vi "DllFxpPolarToRectTemp.vi"(6 "ready for output":bool, 8 "input valid":bool, 10 "phase":fxp<+/-,64,32>, 11 "magnitude":fxp<+/-,64,32>) -> (0 "output valid":bool, 2 "y":fxp<+,1,1>, 3 "x":fxp<+,1,1>, 4 "ready for input":bool)   [LabVIEW 2017]
uses:
  <vilib>/rvi/FXPMathLib/FxpPolarToRect/subVIs/nifxpmath_PolarToRect_SimConfig.ctl
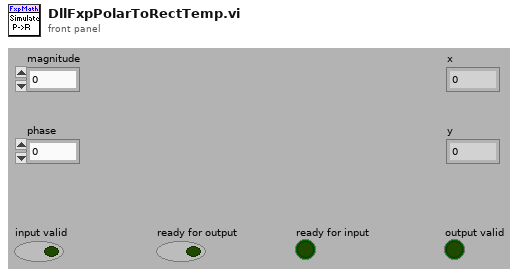
[diagram p1: front panel]
types:
  T1 = typedef "nifxpmath_PolarToRect_SimConfig.ctl" = cluster{"kXYLen":u16, "kPhaseLen":u16, "kPhaseIwl":i16, "kPhaseSigned":bool, "kMagnitudeLen":u16, "kMagnitudeSigned":bool, "kGainCompst":bool, "kCoarseRotation":bool, "kPrecision":u16, "kIteration":u16, "kQuaMode":u16, "HandShake":bool, "InputRegister":bool, "OutputRegister":bool, "CycleLimit":u16, "StrictLimit":bool, "PrescaleCycle":bool}
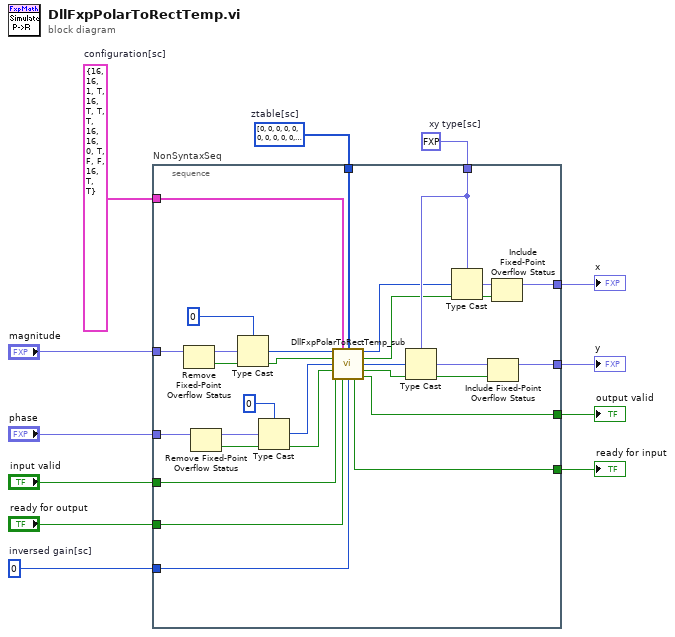
[diagram p0: block diagram]
diagram:
  w1 = T1 {"kXYLen"=16, "kPhaseLen"=16, "kPhaseIwl"=1, "kPhaseSigned"=TRUE, "kMagnitudeLen"=16, "kMagnitudeSigned"=TRUE, "kGainCompst"=TRUE, "kCoarseRotation"=TRUE, "kPrecision"=16, "kIteration"=16, "kQuaMode"=0, "HandShake"=TRUE, "InputRegister"=FALSE, "OutputRegister"=FALSE, "CycleLimit"=16, "StrictLimit"=TRUE, "PrescaleCycle"=TRUE}  # configuration[sc]
  w8 = fxp<+,1,1> 0.0  # xy type[sc]
  w9 = u64 0  # inversed gain[sc]
  w5 = u64[] [0, 0, 0, 0, 0, 0, 0, 0, 0, 0, 0, 0, 0, 0, 0, 0]  # ztable[sc]
  n1 = stacked-sequence "NonSyntaxSeq" {
    tunnel: "input valid" -> [w28]
    tunnel: w1 -> [w35]
    tunnel: "magnitude" -> [w33]
    tunnel: "phase" -> [w31]
    tunnel: w9 -> [w26]
    tunnel: w8 -> [w38]
    tunnel: [w23] -> w7
    tunnel: [w20] -> w6
    tunnel: w5 -> [w27]
    tunnel: "ready for output" -> [w25]
    tunnel: [w18] -> w3
    tunnel: [w17] -> w2
    frame #0 {
      n2 = Remove Fixed-Point Overflow Status(3:w33) -> (0:w32:bool, 1:w34:fxp<+/-,64,32>)
      n3 = Remove Fixed-Point Overflow Status(3:w31) -> (0:w29:bool, 1:w30:fxp<+/-,64,32>)
      n4 = Type Cast(type=u64 0, x=w34) -> (*(type *) &x=w16:u64)
      n5 = Type Cast(type=u64 0, x=w30) -> (*(type *) &x=w15:u64)
      n6 = call <vilib>:"DllFxpPolarToRectTemp_sub.vi"("magnitude"=w16, "configuration[sc]"=w35, "ztable"=w27, "magnitude ovfl status"=w32, "phase"=w15, "phase ovfl status"=w29, "input valid"=w28, "ready for output"=w25, "inversed gain"=w26) -> ("x"=w14:u64, "x ovfl status"=w22:bool, "y"=w13:u64, "y ovfl status"=w19:bool, "ready for input"=w17:bool, "output valid"=w18:bool)  [unwired: 1 out]
      n7 = Type Cast(type=w38, x=w13) -> (*(type *) &x=w21:fxp<+,1,1>)
      n8 = Type Cast(type=w38, x=w14) -> (*(type *) &x=w24:fxp<+,1,1>)
      n9 = Include Fixed-Point Overflow Status(2:w19, 3:w21) -> (1:w20:fxp<+,1,1>)
      n10 = Include Fixed-Point Overflow Status(2:w22, 3:w24) -> (1:w23:fxp<+,1,1>)
    }
  }
  "output valid" <- w3
  "ready for input" <- w2
  "x" <- w7
  "y" <- w6
